vi "Method1.vi"(9 "Body Data":string, 10 "Form Data":cluster{"key":string[], "value":string[]}, 11 "Method":string) -> (3 "Content":string)   [LabVIEW 2019, in "HTTP Server.lvlib"]
uses:
  HTTP Server.lvlib
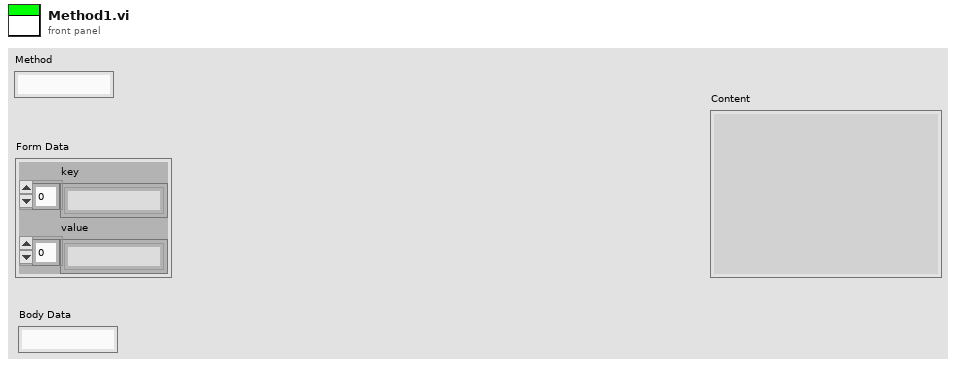
[diagram p1: front panel]
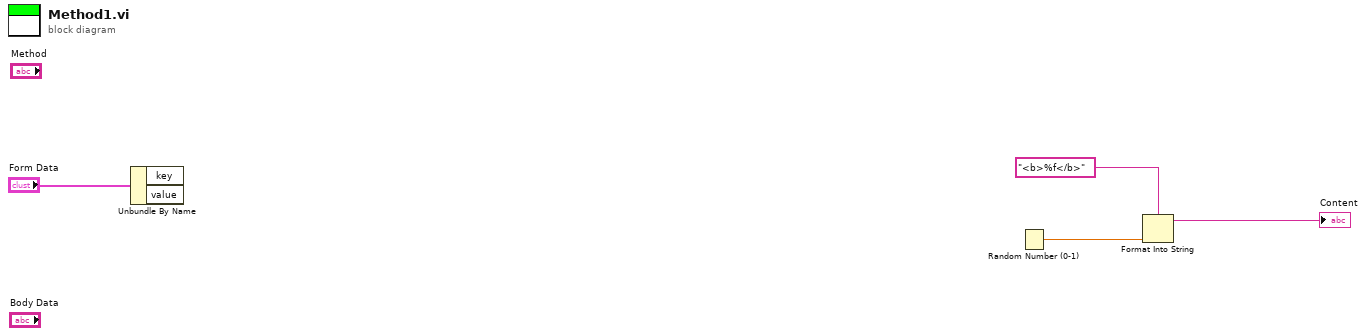
[diagram p0: block diagram]
diagram:
  n1 = Unbundle By Name("Form Data") -> ()  [unwired: 2 out]
  n2 = Random Number (0-1)() -> (number: 0 to 1=w2:dbl)
  n3 = Format Into String(format string="<b>%f</b>" ("Content"), w2) -> (resulting string=→"Content":string)  [unwired: 2 in, 1 out]
